vi "Is New Trial - stim. gen. loop.vi"(1 "Position data":dbl, 2 "Minimum value drop":dbl=-50.0) -> (0 "Boolean":bool)   [LabVIEW 2017]
panel:
  out "Numeric":dbl
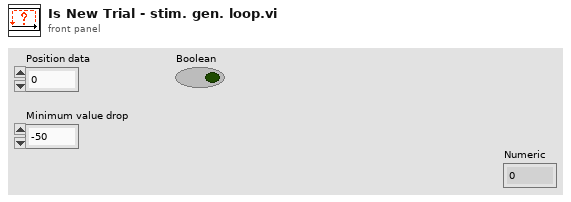
[diagram p1: front panel]
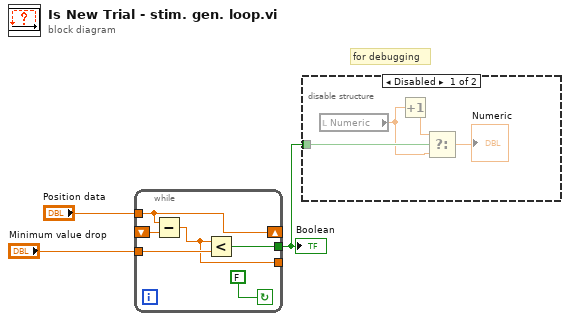
[diagram p0: block diagram]
diagram:
  # "for debugging"
  n1 = while {
    shift-left: _ -> [w7]
    shift-right: [w8] -> _
    tunnel: "Position data" -> [w8]
    tunnel: "Minimum value drop" -> [w6]
    tunnel: [w5] -> w1
    tunnel: [w4] -> _
    stop <- FALSE continue-if-true
    n2 = Subtract(x=w8, y=w7) -> (x-y=w4:dbl)
    n3 = Less?(x=w4, y=w6) -> (x < y?=w5:bool)
  }
  "Boolean" <- w1
  n4 = disable-structure shown="Disabled" {
    disable-tunnel: w1 -> [w13 _]
    frame Disabled {
      n5 = local read "Numeric"() -> (w10:dbl)
      n6 = Increment(x=w10) -> (x+1=w11:dbl)
      n7 = Select(t=w11, s=w13, f=w10) -> (s? t:f=→"Numeric":dbl)
    }
    frame Enabled {
    }
  }
